vi "Msg.vi"(7 "jettl in":refnum<class "jettl.lvclass">, 11 "Teardown Msg Strategy in":refnum<class "Teardown Msg Strategy.lvclass">) -> (5 "jettl out":refnum<class "jettl.lvclass">)   [LabVIEW 2021, in "jettl Msg Teardown.lvlib" / "Teardown Msg Strategy.lvclass"]
uses:
  Teardown Msg Strategy.lvclass
  jettl/jettl/jettl.lvclass
  jettl Msg Teardown/jettl Msg Teardown.lvclass
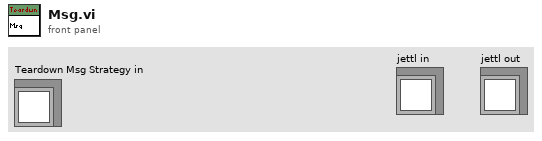
[diagram p1: front panel]
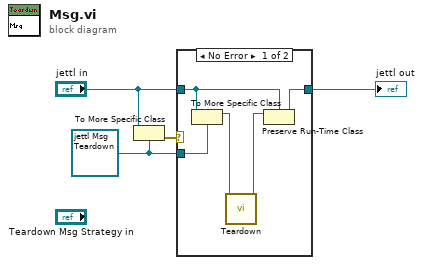
[diagram p0: block diagram]
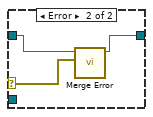
[diagram p2: hidden frame]
diagram:
  w3 = refnum<class "jettl Msg Teardown.lvclass"> refnum ("Destroy.lvlib:Destroy.lvclass")
  n1 = To More Specific Class(target class=w3, reference="jettl in") -> (error out=w4:errorcluster)  [unwired: 1 in, 1 out]
  n2 = case shown="No Error" w4 {
    selector: w4 -> [_ w10]
    tunnel: [w7 w11] -> w1
    tunnel: "jettl in" -> [w8 w12]
    tunnel: w3 -> [w9 _]
    frame No Error {
      n3 = To More Specific Class(target class=w9, reference=w8) -> (specific class reference=w6:refnum<class "jettl Msg Teardown.lvclass">)  [unwired: 1 in, 1 out]
      n4 = call-dynamic "Teardown.vi"("jettl Msg Teardown in"=w6) -> ("jettl Msg Teardown out"=w5:refnum<class "jettl Msg Teardown.lvclass">)  [unwired: 10 in]
      n5 = Preserve Run-Time Class(object in=w5, 2:w8) -> (object out=w7:refnum<class "jettl.lvclass">)  [unwired: 1 in, 1 out]
    }
    frame Error {
      n6 = call-dynamic "Merge Error.vi"("Error"=w10, "Merge Error in"=w12) -> ("Merge Error out"=w11:refnum<class "jettl.lvclass">)  [unwired: 9 in]
    }
  }
  "jettl out" <- w1
